vi "CloseCamera.vi"(8 "error in (no error)":errorcluster, 11 "Photometrics Cam v2 in":refnum<class "Photometrics_CH-250_Cam.lvclass">) -> (0 "error out":errorcluster, 3 "Photometrics Cam v2 Out":refnum<class "Photometrics_CH-250_Cam.lvclass">)   [LabVIEW 2013, in "Photometrics_CH-250_Cam.lvclass"]
uses:
  Photometrics_CH-250_Cam.lvclass
  CameraSessionClass/CS250-CameraHardwareClass.lvclass
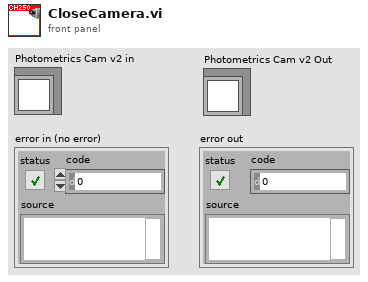
[diagram p1: front panel]
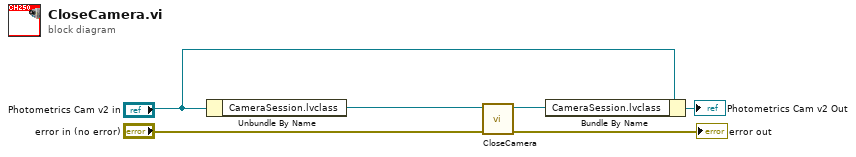
[diagram p0: block diagram]
diagram:
  n1 = Unbundle By Name("Photometrics Cam v2 in") -> ("CameraSession.lvclass"=w5:refnum<class "CS250-CameraHardwareClass.lvclass">)
  n2 = call-dynamic "CloseCamera.vi"("error in (no error)"="error in (no error)", "CameraSession in"=w5) -> ("error out"=→"error out":errorcluster, "CameraSession out"=w2:refnum<class "CS250-CameraHardwareClass.lvclass">)  [unwired: 8 in]
  n3 = Bundle By Name(cluster="Photometrics Cam v2 in", "CameraSession.lvclass"=w2) -> (→"Photometrics Cam v2 Out":refnum<class "Photometrics_CH-250_Cam.lvclass">)
